vi "SubModule Config.vi"(6 "Status":bool, 8 "error in (no error)":errorcluster, 9 "Cycles":i32, 10 "Name":string, 11 "Nikon in":refnum<class "Nikon.lvclass">) -> (0 "error out":errorcluster, 3 "Nikon out":refnum<class "Nikon.lvclass">)   [LabVIEW 2021, in "Nikon.lvclass"]
uses:
  Nikon.lvclass
  C:/Projects/InstrPanel/Classes/Camera/Camera.lvclass
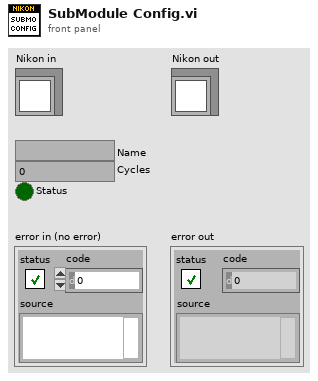
[diagram p1: front panel]
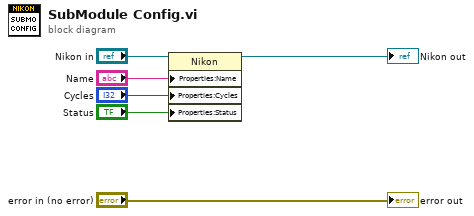
[diagram p0: block diagram]
diagram:
  n1 = property class="Nikon"(reference="Nikon in", "Properties:Name"="Name", "Properties:Cycles"="Cycles", "Properties:Status"="Status") -> (reference out=→"Nikon out":refnum<class "Nikon.lvclass">)  [unwired: 1 in, 1 out]
  "error out" <- "error in (no error)"
